vi "Data checking (SILAR).vi"(0 "Необходимое кол-во циклов":i32=2, 1 "Режим погружения подложки":u16(ring)=1 items=["Частичное", "Полное"], 3 "Подъема подложки над раствором":dbl[](array[numeric])=[2.9, 2.9, 2.9, 2.9], 4 "Подъема подложки из раствора":dbl[](array[numeric])=[1.33, 1.33, 0.0, 0.0], 5 "Кол-во используемых растворов":i32(ring)=2 items=["Один"=1, "Два"=2, "Три"=3, "Четыре"=4], 6 "Время нахождения в растворе (секунды)":dbl[](array[numeric])=[2.0, 1.0, 2.0, 1.0], 7 "Необходимая температура":dbl[](array[numeric])=[38.0, 40.0, 42.0, 44.0], 8 "Высота стакана":dbl, 9 "Кол-во погружений в каждый стакан за один цикл":i32[](array[numeric])=[1, 1, 0, 0], 10 "Задержки после подъема из раствора":dbl[](array[numeric])=[1.0, 1.0, 1.0, 1.0], 11 "Опускания подложки в раствор":dbl[](array[numeric])=[1.33, 1.33, 0.0, 0.0], 12 "Глубина погружения в раствор":dbl[](array[numeric])=[55.0, 55.0, 55.0, 55.0], 13 "Опускания подложки до раствора":dbl[](array[numeric])=[2.9, 2.9, 2.9, 2.9], 14 "Высота подложки":dbl, 15 "Кол-во жидкости в каждом стакане (мм)":dbl[](array[numeric])=[55.0, 55.0, 55.0, 55.0]) -> (2 "ПРОВЕРКА":i16)   [LabVIEW 2016]
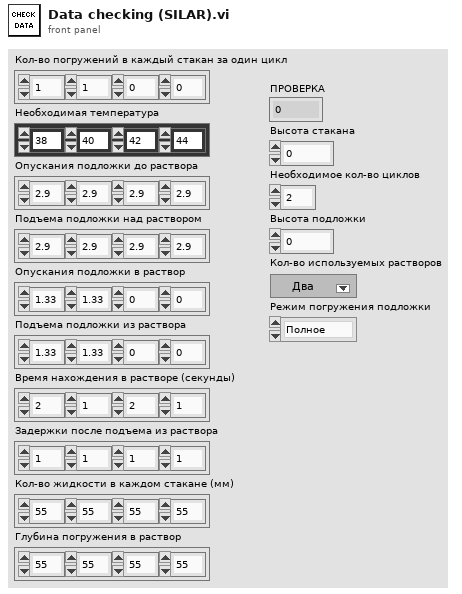
[diagram p1: front panel]
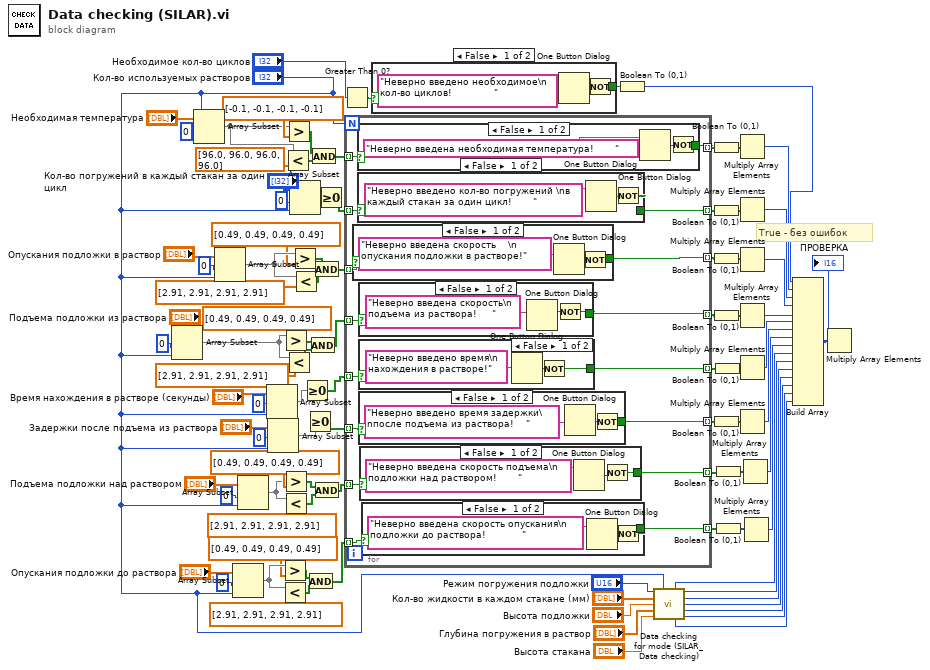
[diagram p0: block diagram]
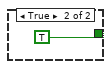
[diagram p2: hidden frame]
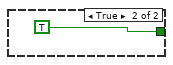
[diagram p3: hidden frame]
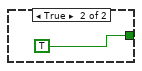
[diagram p4: hidden frame]
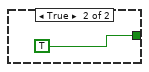
[diagram p5: hidden frame]
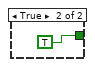
[diagram p6: hidden frame]
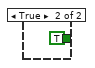
[diagram p7: hidden frame]
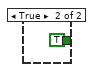
[diagram p8: hidden frame]
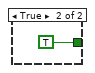
[diagram p9: hidden frame]
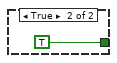
[diagram p10: hidden frame]
diagram:
  # "True - без ошибок"
  n1 = Array Subset(array="Подъема подложки из раствора", index=0, length="Кол-во используемых растворов") -> (w42:dbl[])
  n2 = Array Subset(array="Необходимая температура", index=0, length="Кол-во используемых растворов") -> (w29:dbl[])
  n3 = Array Subset(array="Опускания подложки в раствор", index=0, length="Кол-во используемых растворов") -> (w45:dbl[])
  n4 = Array Subset(array="Опускания подложки до раствора", index=0, length="Кол-во используемых растворов") -> (w39:dbl[])
  n5 = Array Subset(array="Подъема подложки над раствором", index=0, length="Кол-во используемых растворов") -> (w19:dbl[])
  n6 = Array Subset(array="Время нахождения в растворе (секунды)", index=0, length="Кол-во используемых растворов") -> (w47:dbl[])
  n7 = Array Subset(array="Задержки после подъема из раствора", index=0, length="Кол-во используемых растворов") -> (w82:dbl[])
  n8 = Greater?(x=w39, y=dbl[] [0.49, 0.49, 0.49, 0.49]) -> (0:w38:bool[])
  n9 = Less?(x=w39, y=dbl[] [2.91, 2.91, 2.91, 2.91]) -> (x < y?=w58:bool[])
  n10 = Greater?(x=w42, y=dbl[] [0.49, 0.49, 0.49, 0.49]) -> (0:w40:bool[])
  n11 = Greater?(x=w19, y=dbl[] [0.49, 0.49, 0.49, 0.49]) -> (0:w36:bool[])
  n12 = Less?(x=w19, y=dbl[] [2.91, 2.91, 2.91, 2.91]) -> (x < y?=w62:bool[])
  n13 = Less?(x=w29, y=dbl[] [96.0, 96.0, 96.0, 96.0]) -> (x < y?=w30:bool[])
  n14 = Greater?(x=w29, y=dbl[] [-0.1, -0.1, -0.1, -0.1]) -> (0:w31:bool[])
  n15 = Less?(x=w42, y=dbl[] [2.91, 2.91, 2.91, 2.91]) -> (x < y?=w48:bool[])
  n16 = Array Subset(array="Кол-во погружений в каждый стакан за один цикл", index=0, length="Кол-во используемых растворов") -> (w50:i32[])
  n17 = Greater?(x=w45, y=dbl[] [0.49, 0.49, 0.49, 0.49]) -> (0:w43:bool[])
  n18 = Less?(x=w45, y=dbl[] [2.91, 2.91, 2.91, 2.91]) -> (x < y?=w80:bool[])
  n19 = Greater Or Equal To 0?(x=w47) -> (x >= 0?=w46:bool[])
  n20 = Greater Or Equal To 0?(x=w82) -> (x >= 0?=w79:bool[])
  n21 = And(x=w38, y=w58) -> (x .and. y?=w55:bool[])
  n22 = And(x=w40, y=w48) -> (x .and. y?=w78:bool[])
  n23 = And(x=w31, y=w30) -> (x .and. y?=w27:bool[])
  n24 = And(x=w43, y=w80) -> (x .and. y?=w77:bool[])
  n25 = And(x=w36, y=w62) -> (x .and. y?=w56:bool[])
  n26 = Greater Or Equal To 0?(x=w50) -> (x >= 0?=w49:bool[])
  n27 = Greater Than 0?(x="Необходимое кол-во циклов") -> (x > 0?=w81:bool)
  n28 = for {
    N: "Кол-во используемых растворов" -> [_]
    tunnel: w49 -> [w111] mode=indexing
    tunnel: w79 -> [w110] mode=indexing
    tunnel: w46 -> [w109] mode=indexing
    tunnel: w78 -> [w108] mode=indexing
    tunnel: w77 -> [w107] mode=indexing
    tunnel: [w106] -> w76 mode=indexing
    tunnel: [w105] -> w75 mode=indexing
    tunnel: [w104] -> w73 mode=indexing
    tunnel: [w103] -> w72 mode=indexing
    tunnel: [w102] -> w69 mode=indexing
    tunnel: w56 -> [w101] mode=indexing
    tunnel: w55 -> [w100] mode=indexing
    tunnel: [w99] -> w52 mode=indexing
    tunnel: [w98] -> w51 mode=indexing
    tunnel: w27 -> [w97] mode=indexing
    tunnel: [w96] -> w26 mode=indexing
    n29 = case shown="False" w107 {
      tunnel: [w136 TRUE] -> w102
      frame False {
        n30 = One Button Dialog(message="Неверно введена скорость    \n опускания подложки в растворе!") -> (true=w137:bool)  [unwired: 1 in]
        n31 = Not(x=w137) -> (.not. x?=w136:bool)
      }
      frame True {
      }
    }
    n32 = case shown="False" w97 {
      tunnel: [w112 TRUE] -> w96
      frame False {
        n33 = One Button Dialog(message="Неверно введена необходимая температура!       ") -> (true=w113:bool)  [unwired: 1 in]
        n34 = Not(x=w113) -> (.not. x?=w112:bool)
      }
      frame True {
      }
    }
    n35 = case shown="False" w111 {
      tunnel: [w140 TRUE] -> w106
      frame False {
        n36 = One Button Dialog(message="Неверно введено кол-во погружений \nв каждый стакан за один цикл!       ") -> (true=w141:bool)  [unwired: 1 in]
        n37 = Not(x=w141) -> (.not. x?=w140:bool)
      }
      frame True {
      }
    }
    n38 = case shown="False" w108 {
      tunnel: [w132 TRUE] -> w103
      frame False {
        n39 = One Button Dialog(message="Неверно введена скорость\n  подъема из раствора!     ") -> (true=w133:bool)  [unwired: 1 in]
        n40 = Not(x=w133) -> (.not. x?=w132:bool)
      }
      frame True {
      }
    }
    n41 = case shown="False" w109 {
      tunnel: [w128 TRUE] -> w104
      frame False {
        n42 = One Button Dialog(message="Неверно введено время\n нахождения в растворе!") -> (true=w129:bool)  [unwired: 1 in]
        n43 = Not(x=w129) -> (.not. x?=w128:bool)
      }
      frame True {
      }
    }
    n44 = case shown="False" w110 {
      tunnel: [w124 TRUE] -> w105
      frame False {
        n45 = One Button Dialog(message="Неверно введено время задержки\nпосле подъема из раствора!    ") -> (true=w125:bool)  [unwired: 1 in]
        n46 = Not(x=w125) -> (.not. x?=w124:bool)
      }
      frame True {
      }
    }
    n47 = case shown="False" w101 {
      tunnel: [w120 TRUE] -> w98
      frame False {
        n48 = One Button Dialog(message="Неверно введена скорость подъема\n подложки над раствором!       ") -> (true=w121:bool)  [unwired: 1 in]
        n49 = Not(x=w121) -> (.not. x?=w120:bool)
      }
      frame True {
      }
    }
    n50 = case shown="False" w100 {
      tunnel: [w116 TRUE] -> w99
      frame False {
        n51 = One Button Dialog(message="Неверно введена скорость опускания\n подложки до раствора!            ") -> (true=w117:bool)  [unwired: 1 in]
        n52 = Not(x=w117) -> (.not. x?=w116:bool)
      }
      frame True {
      }
    }
  }
  n53 = case shown="False" w81 {
    tunnel: [w144 TRUE] -> w68
    frame False {
      n54 = One Button Dialog(message="Неверно введено необходимое\n кол-во циклов!              ") -> (true=w145:bool)  [unwired: 1 in]
      n55 = Not(x=w145) -> (.not. x?=w144:bool)
    }
    frame True {
    }
  }
  n56 = Boolean To (0,1)(Boolean=w68) -> (0, 1=w17:i16)
  n57 = call "Data checking for mode (SILAR_Data checking).vi"("Режим погружения подложки"="Режим погружения подложки", "Кол-во используемых растворов"="Кол-во используемых растворов", "Кол-во жидкости в каждом стакане (мм)"="Кол-во жидкости в каждом стакане (мм)", "Высота подложки"="Высота подложки", "Глубина погружения в раствор"="Глубина погружения в раствор", "Высота стакана"="Высота стакана") -> ("1"=w7:i16, "2"=w6:i16, "3"=w5:i16, "4"=w4:i16, "5"=w3:i16, "7"=w1:i16, "6"=w2:i16)  [unwired: 3 in]
  n58 = Boolean To (0,1)(Boolean=w26) -> (0, 1=w25:i16[])
  n59 = Boolean To (0,1)(Boolean=w76) -> (0, 1=w67:i16[])
  n60 = Boolean To (0,1)(Boolean=w69) -> (0, 1=w70:i16[])
  n61 = Boolean To (0,1)(Boolean=w72) -> (0, 1=w71:i16[])
  n62 = Boolean To (0,1)(Boolean=w75) -> (0, 1=w74:i16[])
  n63 = Boolean To (0,1)(Boolean=w73) -> (0, 1=w11:i16[])
  n64 = Boolean To (0,1)(Boolean=w51) -> (0, 1=w54:i16[])
  n65 = Boolean To (0,1)(Boolean=w52) -> (0, 1=w53:i16[])
  n66 = Multiply Array Elements(1:w25) -> (0:w16:i16)
  n67 = Multiply Array Elements(1:w67) -> (0:w15:i16)
  n68 = Multiply Array Elements(1:w70) -> (0:w14:i16)
  n69 = Multiply Array Elements(1:w71) -> (0:w13:i16)
  n70 = Multiply Array Elements(1:w11) -> (0:w12:i16)
  n71 = Multiply Array Elements(1:w74) -> (0:w10:i16)
  n72 = Multiply Array Elements(1:w54) -> (0:w9:i16)
  n73 = Multiply Array Elements(1:w53) -> (0:w8:i16)
  n74 = Build Array(w17, w16, w15, w14, w13, w12, w10, w9, w8, w7, w6, w5, w4, w3, w2, w1) -> (w66:i16[])
  n75 = Multiply Array Elements(1:w66) -> (0:→"ПРОВЕРКА":i16)
